vi "Create Test Node File.vi"(8 "error in (no error)":errorcluster, 10 "Item Configurations":refnum<class "Item Configuration.lvclass">[](array[class]), 11 "Test Node Project Path":path) -> (0 "error out":errorcluster)   [LabVIEW 2013, in "File IO.lvlib"]
uses:
  File IO.lvlib
  Item Configuration/Item Configuration/Item Configuration.lvclass
  <vilib>/xml/Load XML String.vi
  <vilib>/xml/Close Reference(Node).vi
  <vilib>/xml/NI_XML.lvlib
  <resource>/objmgr/DOMUserDefRef.rc
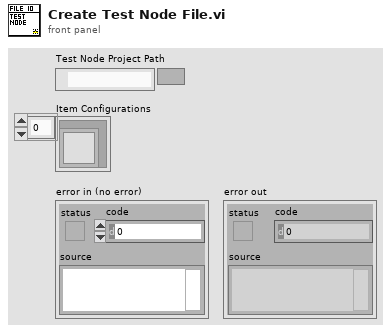
[diagram p1: front panel]
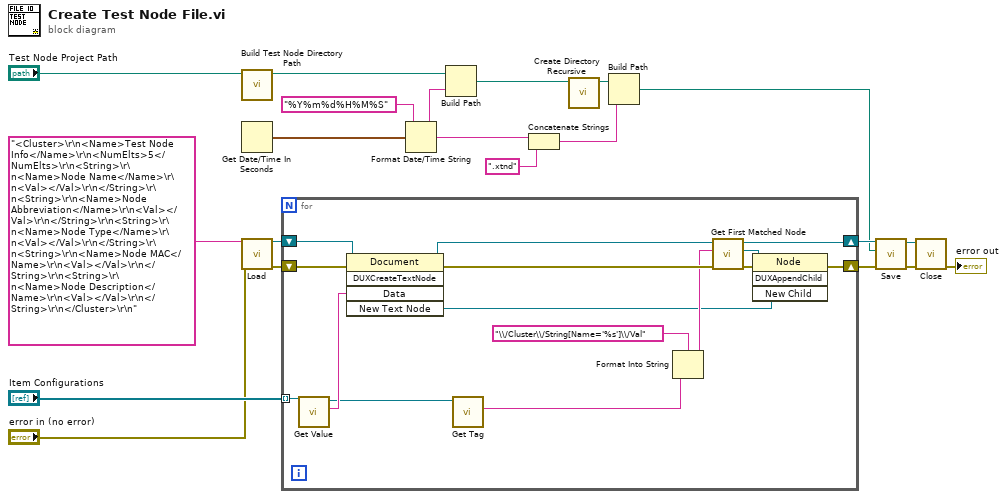
[diagram p0: block diagram]
diagram:
  n1 = call "Build Test Node Directory Path.vi"("Project Path"="Test Node Project Path") -> ("Test Node Directory Path"=w4:path)  [unwired: 10 in]
  n2 = Get Date/Time In Seconds() -> (seconds since 1Jan1904=w3:timestamp)
  n3 = call-poly <vilib>:"Load.vi"("XML string"="<Cluster>\r\n<Name>Test Node Info</Name>\r\n<NumElts>5</NumElts>\r\n<String>\r\n<Name>Node Name</Name>\r\n<Val></Val>\r\n</String>\r\n<String>\r\n<Name>Node Abbreviation</Name>\r\n<Val></Val>\r\n</String>\r\n<String>\r\n<Name>Node Type</Name>\r\n<Val></Val>\r\n</String>\r\n<String>\r\n<Name>Node MAC</Name>\r\n<Val></Val>\r\n</String>\r\n<String>\r\n<Name>Node Description</Name>\r\n<Val></Val>\r\n</String>\r\n</Cluster>\r\n" ("xml string"), "error in (no error)"="error in (no error)") -> ("DOM document out"=w20:refnum<k20>, "error out"=w19:errorcluster)  [unwired: 11 in, 1 out]
  n4 = for {
    shift-right: [w35] -> w16
    shift-left: w20 -> [w32]
    shift-right: [w28] -> w15
    shift-left: w19 -> [w31]
    tunnel: "Item Configurations" -> [w27] mode=indexing
    n5 = call-dynamic "Get Value.vi"("Item Configuration in"=w27) -> ("Project Info Value"=w26:string, "Item Configuration out"=w23:refnum<class "Item Configuration.lvclass">)  [unwired: 8 in, 1 out]
    n6 = invoke class="Document" method="DUXCreateTextNode"(reference=w32, error in=w31, "Data"=w26) -> (reference out=w33:refnum<k20>, error out=w30:errorcluster, "New Text Node"=w21:refnum<k20>)  [unwired: 2 in, 2 out]
    n7 = call-dynamic "Get Tag.vi"("Item Configuration in"=w23) -> ("Project Info Tag"=w24:string)  [unwired: 8 in, 2 out]
    n8 = Format Into String(format string="\\/Cluster\\/String[Name='%s']\\/Val" ("XPath expression"), w24) -> (resulting string=w22:string)  [unwired: 2 in, 1 out]
    n9 = call <vilib>:"Get First Matched Node.vi"("error in (no error)"=w30, "XPath expression"=w22, "node in"=w33) -> ("error out"=w29:errorcluster, "node result"=w34:refnum<k20>, "node out"=w35:refnum<k20>)  [unwired: 6 in]
    n10 = invoke class="Node" method="DUXAppendChild"(reference=w34, error in=w29, "New Child"=w21) -> (error out=w28:errorcluster)  [unwired: 1 in, 3 out]
  }
  n11 = Format Date/Time String(time format string (%c)="%Y%m%d%H%M%S", seconds (now)=w3) -> (date/time string=w1:string)  [unwired: 1 in]
  n12 = Build Path(base path=w4, name or relative path=w1) -> (appended path=w9:path)
  n13 = Concatenate Strings(w1, ".xtnd" ("string")) -> (w7:string)
  n14 = call <vilib>:"Create Directory Recursive.vi"("directory"=w9) -> ("directory copy"=w8:path)  [unwired: 4 in, 2 out]
  n15 = Build Path(base path=w8, name or relative path=w7) -> (appended path=w2:path)
  n16 = call <vilib>:"Save.vi"("error in (no error)"=w15, "XML file path"=w2, "DOM document in"=w16) -> ("error out"=w13:errorcluster, "DOM document out"=w14:refnum<k20>)  [unwired: 6 in, 1 out]
  n17 = call-poly <vilib>:"Close.vi"("error in (no error)"=w13, "node"=w14) -> ("error out"=→"error out":errorcluster)  [unwired: 7 in]
